vi "切换射频开关.vi"(8 "error in":errorcluster caption="error constant", 9 "COM":u16, 11 "A":u16) -> (0 "error out":errorcluster caption="error constant", 1 "ask":string, 2 "Isfailed":bool)   [LabVIEW 2015]
uses:
  Global/SeverGlobal.vi
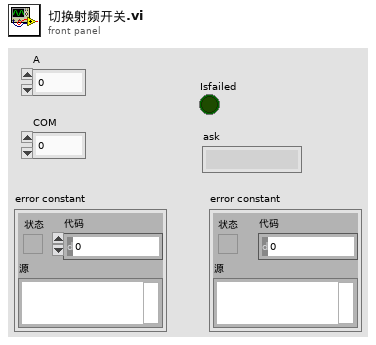
[diagram p1: front panel]
types:
  T1 = enum16{"Standard", "Buffered", "CRLF", "Immediate"}
  T2 = cluster{"IP_A":string, "PORT_A":i32, "IP_B":string, "PORT_B":i32, "IP_CLK":string, "PORT_CLK":i32, "IP_SWITCH":string, "PORT_SWITCH":i32}
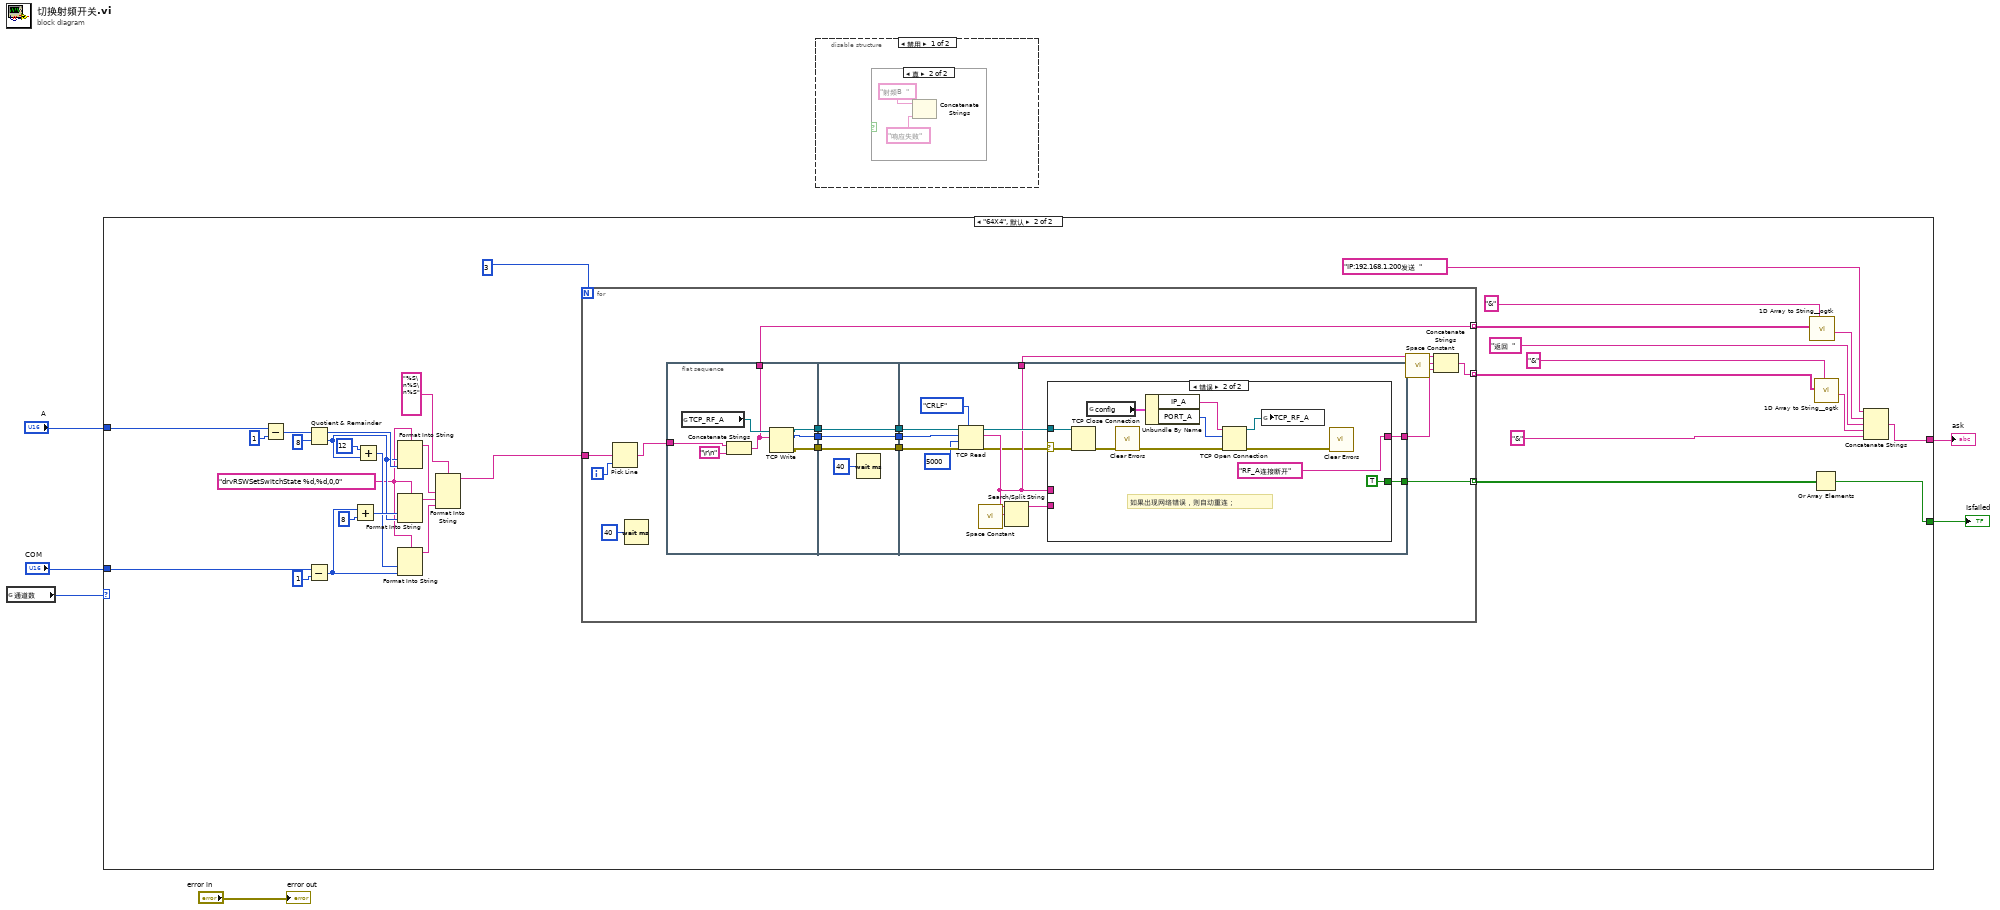
[diagram p0: block diagram]
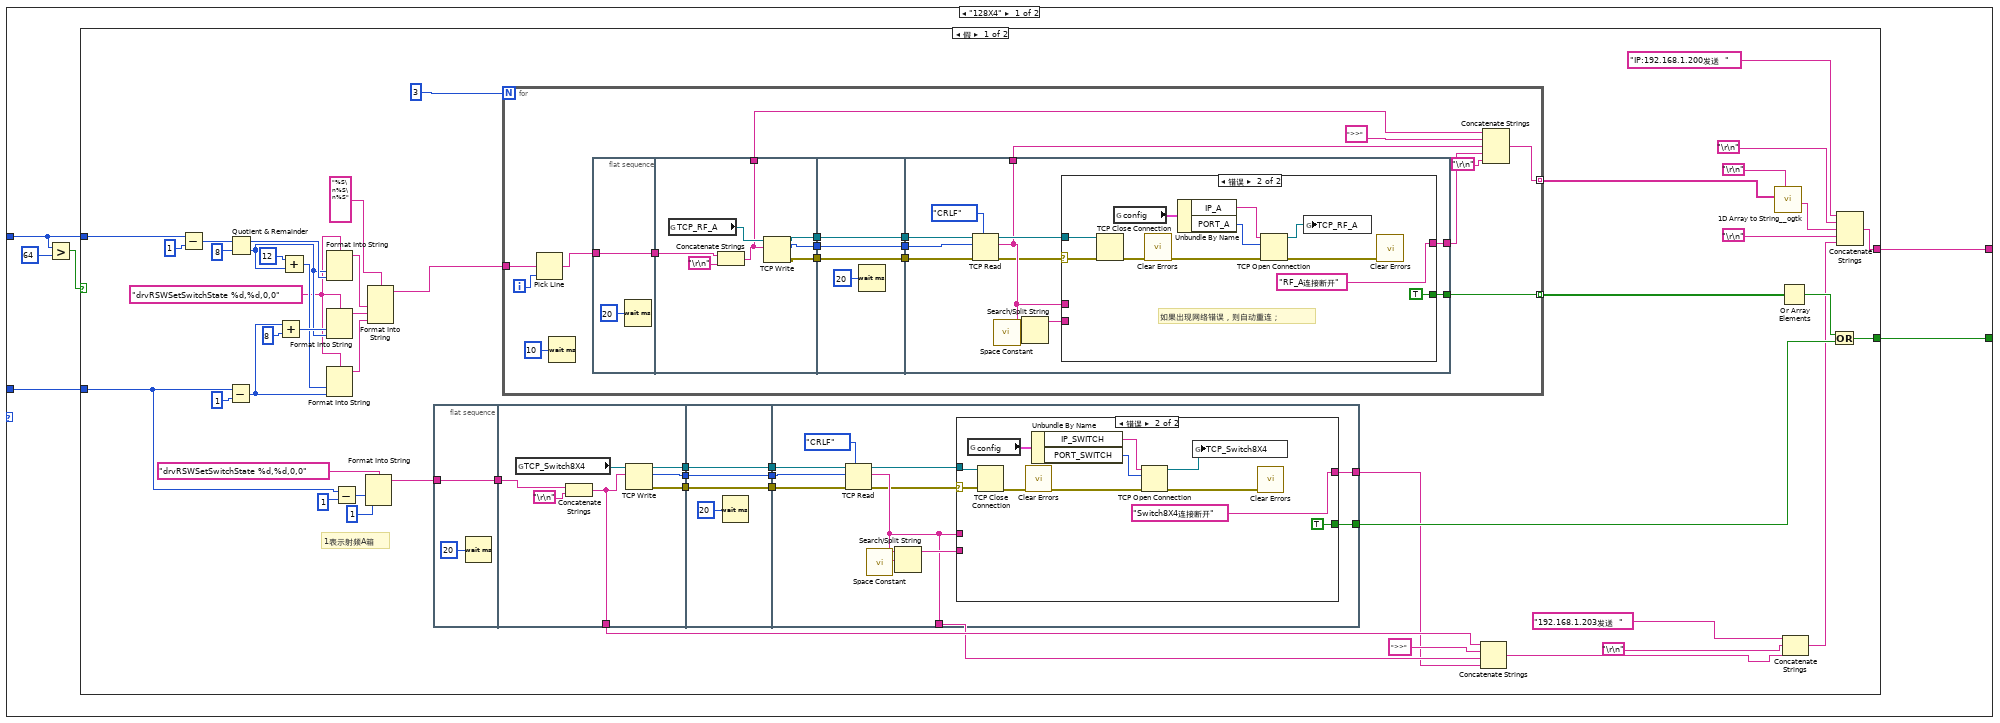
[diagram p2: hidden frame]
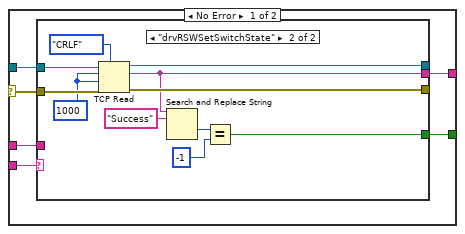
[diagram p3: hidden frame]
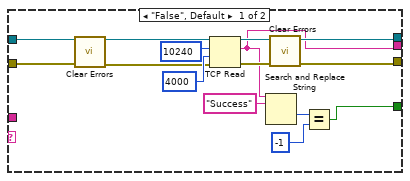
[diagram p4: hidden frame]
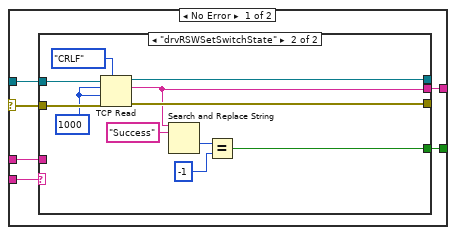
[diagram p5: hidden frame]
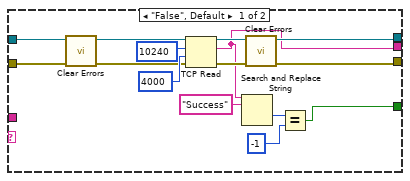
[diagram p6: hidden frame]
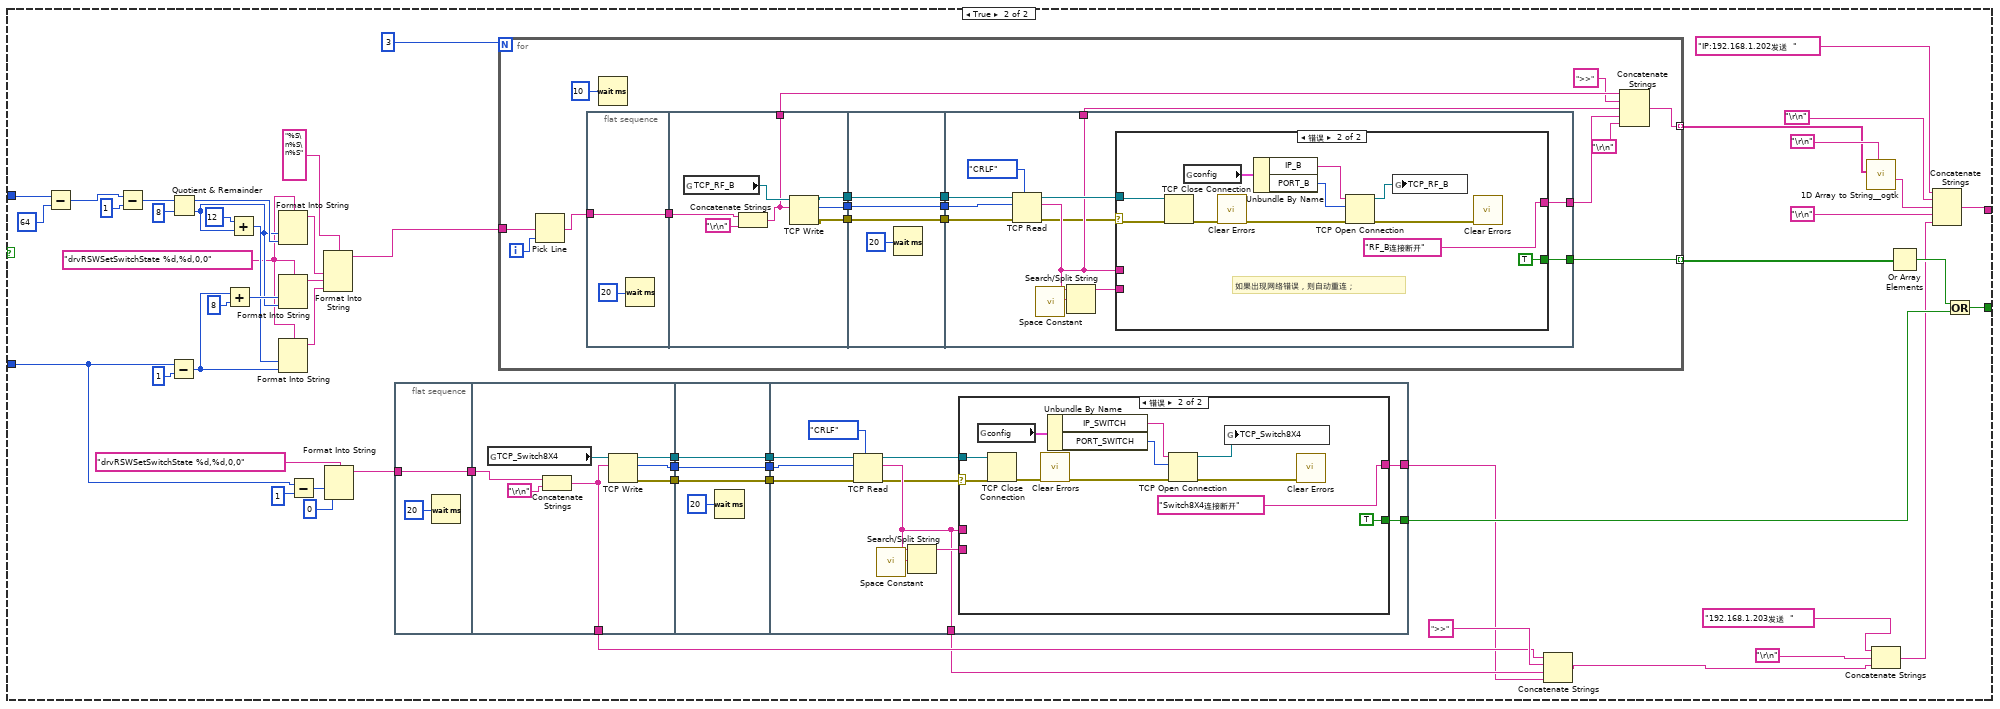
[diagram p7: hidden frame]
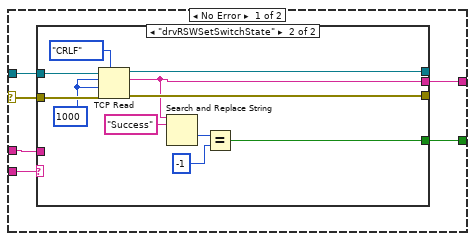
[diagram p8: hidden frame]
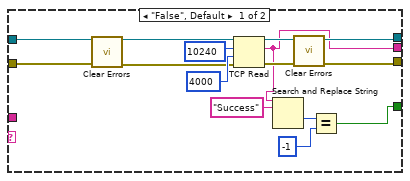
[diagram p9: hidden frame]
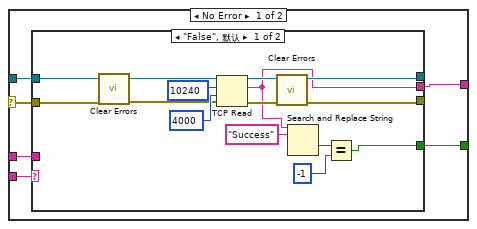
[diagram p10: hidden frame]
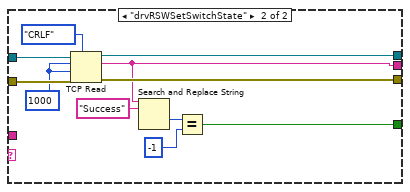
[diagram p11: hidden frame]
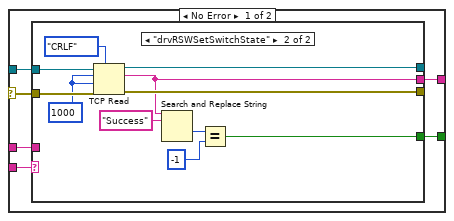
[diagram p12: hidden frame]
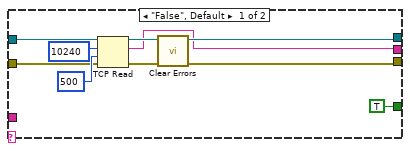
[diagram p13: hidden frame]
diagram:
  n1 = global read "SeverGlobal.vi" "通道数"() -> (w2:enum16{"64X4", "128X4"})
  n2 = case shown="\"64X4\", 默认" w2 {
    tunnel: "A" -> [w12 w444]
    tunnel: "COM" -> [w9 w443]
    tunnel: [w8 w423] -> w3
    tunnel: [w7 w413] -> w1
    frame "128X4" {
      n3 = Greater?(x=w12, y=u16 64) -> (0:w10:bool)
      n4 = case shown="假" w10 {
        tunnel: w12 -> [w45 w246]
        tunnel: w9 -> [w41 w232]
        tunnel: [w29 w229] -> w8
        tunnel: [w26 w218] -> w7
        frame False {
          w48 = "drvRSWSetSwitchState %d,%d,0,0" ("格式字符串")
          # "1表示射频A箱"
          n5 = Subtract(x=w45, y=1) -> (x-y=w62:i32)
          n6 = Subtract(x=w41, y=1) -> (x-y=w53:i32)
          n7 = Quotient & Remainder(x=w62, y=8) -> (x-y*floor(x/y)=w57:i32, floor(x/y)=w55:i32)
          n8 = Add(x=w53, y=8) -> (x+y=w56:i32)
          n9 = Add(x=12, y=w55) -> (x+y=w54:i32)
          n10 = Format Into String(format string=w48, w55, w57) -> (resulting string=w51:string)  [unwired: 2 in, 1 out]
          n11 = Format Into String(format string=w48, w56, w55) -> (resulting string=w50:string)  [unwired: 2 in, 1 out]
          n12 = Format Into String(format string=w48, w54, w53) -> (resulting string=w49:string)  [unwired: 2 in, 1 out]
          n13 = Subtract(x=w41, y=1) -> (x-y=w44:i32)
          n14 = Format Into String(format string="drvRSWSetSwitchState %d,%d,0,0" ("格式字符串"), w44, i16 1 ("input 2")) -> (resulting string=w39:string)  [unwired: 2 in, 1 out]
          n15 = Format Into String(format string="%S\n%S\n%S", w51, w50, w49) -> (resulting string=w47:string)  [unwired: 2 in, 1 out]
          n16 = flat-sequence {
            tunnel: w39 -> [w65]
            tunnel: [w65] -> w23
            tunnel: [w69] -> w38
            tunnel: [w68] -> w37
            tunnel: [w67] -> w33
            tunnel: [w66] -> w16
            tunnel: w23 -> [w71]
            tunnel: w38 -> [w75]
            tunnel: w37 -> [w74]
            tunnel: [w75] -> w36
            tunnel: [w74] -> w35
            tunnel: [w73] -> w34
            tunnel: w33 -> [w73]
            tunnel: w36 -> [w83]
            tunnel: w35 -> [w82]
            tunnel: w34 -> [w81]
            tunnel: [w80] -> w30
            tunnel: [w79] -> w14
            tunnel: [w78] -> w15
            frame #0 {
              n17 = Wait (ms)(milliseconds to wait=u32 20 ("delay")) -> ()  [unwired: 1 out]
            }
            frame #1 {
              n18 = global read "SeverGlobal.vi" "TCP_Switch8X4"() -> (w72:refnum<k5>)
              n19 = Concatenate Strings(w71, "\r\n") -> (w66:string)
              n20 = TCP Write(connection ID=w72, data in=w66) -> (connection ID out=w69:refnum<k5>, bytes written=w67:i32, error out=w68:errorcluster)  [unwired: 2 in]
            }
            frame #2 {
              n21 = Wait (ms)(milliseconds to wait=u32 20 ("delay")) -> ()  [unwired: 1 out]
            }
            frame #3 {
              n22 = TCP Read(connection ID=w83, bytes to read=w81, error in (no error)=w82, 7:T1."CRLF" ("mode (standard)")) -> (connection ID out=w87:refnum<k5>, data out=w78:string, error out=w77:errorcluster)  [unwired: 1 in]
              n23 = call <vilib>:"Space Constant.vi"() -> ("String"=w84:string)
              n24 = Search/Split String(string=w78, search string/char (-)=w84) -> (substring before match=w86:string)  [unwired: 1 in, 2 out]
              n25 = case shown="错误" w77 {
                selector: w77 -> [w88 w121]
                tunnel: w87 -> [w93 w120]
                tunnel: w86 -> [w92 _]
                tunnel: [w91 TRUE] -> w80
                tunnel: [w90 "Switch8X4连接断开" ("字符串")] -> w79
                tunnel: w78 -> [w89 _]
                frame No Error {
                  n26 = case shown="\"drvRSWSetSwitchState\"" w92 {
                    tunnel: [w102 w116] -> _
                    tunnel: [w101 w115] -> _
                    tunnel: w93 -> [w103 w114]
                    tunnel: w88 -> [w100 w113]
                    tunnel: w89 -> [_ _]
                    tunnel: [w94 w108] -> w91
                    tunnel: [w95 w107] -> w90
                    frame "False", Default {
                      n27 = call <vilib>:"Clear Errors.vi"("error in (no error)"=w100) -> ("error out"=w99:errorcluster)  [unwired: 5 in, 1 out]
                      n28 = TCP Read(connection ID=w103, bytes to read=10240, error in (no error)=w99, 9:4000 ("timeout ms (25000)")) -> (connection ID out=w102:refnum<k5>, data out=w95:string, error out=w105:errorcluster)  [unwired: 1 in]
                      n29 = Search and Replace String(input string=w95, search string="Success") -> (offset past replacement=w96:i32)  [unwired: 6 in, 3 out]
                      n30 = call <vilib>:"Clear Errors.vi"("error in (no error)"=w105) -> ("error out"=w101:errorcluster)  [unwired: 5 in, 1 out]
                      n31 = Equal?(x=w96, y=-1) -> (x = y?=w94:bool)
                    }
                    frame "drvRSWSetSwitchState" {
                      w112 = 1000 ("timeout ms (25000)")
                      n32 = TCP Read(connection ID=w114, bytes to read=w112, error in (no error)=w113, 7:T1."CRLF" ("mode (standard)"), 9:w112) -> (connection ID out=w116:refnum<k5>, data out=w107:string, error out=w115:errorcluster)
                      n33 = Search and Replace String(input string=w107, search string="Success") -> (offset past replacement=w110:i32)  [unwired: 6 in, 3 out]
                      n34 = Equal?(x=w110, y=-1) -> (x = y?=w108:bool)
                    }
                  }
                }
                frame Error {
                  n35 = global read "SeverGlobal.vi" "config"() -> (w124:T2)
                  n36 = TCP Close Connection(connection ID=w120, error in (no error)=w121) -> (error out=w122:errorcluster)  [unwired: 1 in, 1 out]
                  n37 = call <vilib>:"Clear Errors.vi"("error in (no error)"=w122) -> ("error out"=w123:errorcluster)  [unwired: 5 in, 1 out]
                  n38 = Unbundle By Name(w124) -> ("IP_SWITCH"=w125:string, "PORT_SWITCH"=w126:i32)
                  n39 = TCP Open Connection(address=w125, remote port or service name=w126, error in (no error)=w123) -> (connection ID=w127:refnum<k5>, error out=w128:errorcluster)  [unwired: 2 in]
                  n40 = global write "SeverGlobal.vi" "TCP_Switch8X4"(w127) -> ()
                  n41 = call <vilib>:"Clear Errors.vi"("error in (no error)"=w128) -> ()  [unwired: 5 in, 2 out]
                }
              }
            }
          }
          n42 = for {
            N: 3 -> [_]
            tunnel: w47 -> [w146]
            tunnel: [w136] -> w32 mode=indexing
            tunnel: [w133] -> w27 mode=indexing
            i -> [w145]
            n43 = Pick Line(multi-line string=w146, line index=w145) -> (output string=w144:string)  [unwired: 1 in]
            n44 = Wait (ms)(milliseconds to wait=u32 10 ("delay")) -> ()  [unwired: 1 out]
            n45 = flat-sequence {
              tunnel: w144 -> [w148]
              tunnel: [w148] -> w132
              tunnel: [w152] -> w142
              tunnel: [w151] -> w140
              tunnel: [w150] -> w138
              tunnel: [w149] -> w130
              tunnel: w132 -> [w153]
              tunnel: [w158] -> w143
              tunnel: w142 -> [w158]
              tunnel: [w157] -> w141
              tunnel: w140 -> [w157]
              tunnel: [w156] -> w139
              tunnel: w138 -> [w156]
              tunnel: w143 -> [w168]
              tunnel: w141 -> [w167]
              tunnel: w139 -> [w166]
              tunnel: [w163] -> w136
              tunnel: [w162] -> w135
              tunnel: [w161] -> w134
              frame #0 {
                n46 = Wait (ms)(milliseconds to wait=u32 20 ("delay")) -> ()  [unwired: 1 out]
              }
              frame #1 {
                n47 = global read "SeverGlobal.vi" "TCP_RF_A"() -> (w154:refnum<k5>)
                n48 = Concatenate Strings(w153, "\r\n") -> (w149:string)
                n49 = TCP Write(connection ID=w154, data in=w149) -> (connection ID out=w152:refnum<k5>, bytes written=w151:i32, error out=w150:errorcluster)  [unwired: 2 in]
              }
              frame #2 {
                n50 = Wait (ms)(milliseconds to wait=u32 20 ("delay")) -> ()  [unwired: 1 out]
              }
              frame #3 {
                n51 = TCP Read(connection ID=w168, bytes to read=w167, error in (no error)=w166, 7:T1."CRLF" ("mode (standard)")) -> (connection ID out=w164:refnum<k5>, data out=w162:string, error out=w160:errorcluster)  [unwired: 1 in]
                n52 = call <vilib>:"Space Constant.vi"() -> ("String"=w170:string)
                n53 = Search/Split String(string=w162, search string/char (-)=w170) -> (substring before match=w165:string)  [unwired: 1 in, 2 out]
                n54 = case shown="错误" w160 {
                  selector: w160 -> [w171 w210]
                  tunnel: w165 -> [w176 _]
                  tunnel: w164 -> [w175 w211]
                  tunnel: [w174 TRUE] -> w163
                  tunnel: w162 -> [w173 _]
                  tunnel: [w172 "RF_A连接断开" ("字符串")] -> w161
                  frame No Error {
                    n55 = case shown="\"drvRSWSetSwitchState\"" w176 {
                      tunnel: [w185 w199] -> _
                      tunnel: [w184 w198] -> _
                      tunnel: w175 -> [w186 w197]
                      tunnel: w171 -> [w183 w196]
                      tunnel: w173 -> [_ _]
                      tunnel: [w177 w191] -> w174
                      tunnel: [w178 w190] -> w172
                      frame "False", Default {
                        n56 = call <vilib>:"Clear Errors.vi"("error in (no error)"=w183) -> ("error out"=w182:errorcluster)  [unwired: 5 in, 1 out]
                        n57 = TCP Read(connection ID=w186, bytes to read=10240, error in (no error)=w182, 9:4000 ("timeout ms (25000)")) -> (connection ID out=w185:refnum<k5>, data out=w178:string, error out=w188:errorcluster)  [unwired: 1 in]
                        n58 = Search and Replace String(input string=w178, search string="Success") -> (offset past replacement=w181:i32)  [unwired: 6 in, 3 out]
                        n59 = call <vilib>:"Clear Errors.vi"("error in (no error)"=w188) -> ("error out"=w184:errorcluster)  [unwired: 5 in, 1 out]
                        n60 = Equal?(x=w181, y=-1) -> (x = y?=w177:bool)
                      }
                      frame "drvRSWSetSwitchState" {
                        w195 = 1000 ("timeout ms (25000)")
                        n61 = TCP Read(connection ID=w197, bytes to read=w195, error in (no error)=w196, 7:T1."CRLF" ("mode (standard)"), 9:w195) -> (connection ID out=w199:refnum<k5>, data out=w190:string, error out=w198:errorcluster)
                        n62 = Search and Replace String(input string=w190, search string="Success") -> (offset past replacement=w193:i32)  [unwired: 6 in, 3 out]
                        n63 = Equal?(x=w193, y=-1) -> (x = y?=w191:bool)
                      }
                    }
                  }
                  frame Error {
                    # "如果出现网络错误，则自动重连；"
                    n64 = TCP Close Connection(connection ID=w211, error in (no error)=w210) -> (error out=w209:errorcluster)  [unwired: 1 in, 1 out]
                    n65 = global read "SeverGlobal.vi" "config"() -> (w207:T2)
                    n66 = call <vilib>:"Clear Errors.vi"("error in (no error)"=w209) -> ("error out"=w208:errorcluster)  [unwired: 5 in, 1 out]
                    n67 = Unbundle By Name(w207) -> ("IP_A"=w206:string, "PORT_A"=w205:i32)
                    n68 = TCP Open Connection(address=w206, remote port or service name=w205, error in (no error)=w208) -> (connection ID=w204:refnum<k5>, error out=w203:errorcluster)  [unwired: 2 in]
                    n69 = global write "SeverGlobal.vi" "TCP_RF_A"(w204) -> ()
                    n70 = call <vilib>:"Clear Errors.vi"("error in (no error)"=w203) -> ()  [unwired: 5 in, 2 out]
                  }
                }
              }
            }
            n71 = Concatenate Strings(w130, ">>" ("字符串"), w135, w134, "\r\n") -> (w133:string)
          }
          n72 = Concatenate Strings(w16, ">>" ("字符串"), w15, w14) -> (w13:string)
          n73 = call <userlib>:"1D Array to String__ogtk.vi"("delimiter (Tab)"="\r\n", "Array of Strings"=w27) -> ("delimited string"=w28:string)  [unwired: 9 in]
          n74 = Or Array Elements(Boolean array=w32) -> (logical OR=w31:bool)
          n75 = Concatenate Strings("192.168.1.203发送  " ("delimiter (Tab)"), "\r\n", w13) -> (w24:string)
          n76 = Or(x=w31, y=w30) -> (x .or. y?=w29:bool)
          n77 = Concatenate Strings("IP:192.168.1.200发送  " ("delimiter (Tab)"), "\r\n", w28, "\r\n", w24) -> (w26:string)
        }
        frame True {
          w249 = "drvRSWSetSwitchState %d,%d,0,0" ("格式字符串")
          n78 = Subtract(x=w246, y=u16 64) -> (x-y=w244:u16)
          n79 = Subtract(x=w244, y=1) -> (x-y=w263:i32)
          n80 = Subtract(x=w232, y=1) -> (x-y=w254:i32)
          n81 = Quotient & Remainder(x=w263, y=8) -> (x-y*floor(x/y)=w258:i32, floor(x/y)=w256:i32)
          n82 = Add(x=w254, y=8) -> (x+y=w257:i32)
          n83 = Add(x=12, y=w256) -> (x+y=w255:i32)
          n84 = Format Into String(format string=w249, w256, w258) -> (resulting string=w252:string)  [unwired: 2 in, 1 out]
          n85 = Format Into String(format string=w249, w257, w256) -> (resulting string=w251:string)  [unwired: 2 in, 1 out]
          n86 = Format Into String(format string=w249, w255, w254) -> (resulting string=w250:string)  [unwired: 2 in, 1 out]
          n87 = Subtract(x=w232, y=1) -> (x-y=w237:i32)
          n88 = Format Into String(format string="%S\n%S\n%S", w252, w251, w250) -> (resulting string=w248:string)  [unwired: 2 in, 1 out]
          n89 = Format Into String(format string="drvRSWSetSwitchState %d,%d,0,0" ("格式字符串"), w237, i16 0 ("input 2")) -> (resulting string=w233:string)  [unwired: 2 in, 1 out]
          n90 = flat-sequence {
            tunnel: w233 -> [w266]
            tunnel: [w266] -> w226
            tunnel: [w270] -> w243
            tunnel: [w269] -> w242
            tunnel: [w268] -> w241
            tunnel: [w267] -> w216
            tunnel: w226 -> [w272]
            tunnel: w243 -> [w276]
            tunnel: w242 -> [w275]
            tunnel: [w276] -> w240
            tunnel: [w275] -> w239
            tunnel: [w274] -> w238
            tunnel: w241 -> [w274]
            tunnel: w240 -> [w284]
            tunnel: w239 -> [w283]
            tunnel: w238 -> [w282]
            tunnel: [w281] -> w228
            tunnel: [w280] -> w215
            tunnel: [w279] -> w214
            frame #0 {
              n91 = Wait (ms)(milliseconds to wait=u32 20 ("delay")) -> ()  [unwired: 1 out]
            }
            frame #1 {
              n92 = global read "SeverGlobal.vi" "TCP_Switch8X4"() -> (w273:refnum<k5>)
              n93 = Concatenate Strings(w272, "\r\n") -> (w267:string)
              n94 = TCP Write(connection ID=w273, data in=w267) -> (connection ID out=w270:refnum<k5>, bytes written=w268:i32, error out=w269:errorcluster)  [unwired: 2 in]
            }
            frame #2 {
              n95 = Wait (ms)(milliseconds to wait=u32 20 ("delay")) -> ()  [unwired: 1 out]
            }
            frame #3 {
              n96 = TCP Read(connection ID=w284, bytes to read=w282, error in (no error)=w283, 7:T1."CRLF" ("mode (standard)")) -> (connection ID out=w288:refnum<k5>, data out=w280:string, error out=w278:errorcluster)  [unwired: 1 in]
              n97 = call <vilib>:"Space Constant.vi"() -> ("String"=w285:string)
              n98 = Search/Split String(string=w280, search string/char (-)=w285) -> (substring before match=w287:string)  [unwired: 1 in, 2 out]
              n99 = case shown="错误" w278 {
                selector: w278 -> [w289 w322]
                tunnel: w288 -> [w294 w321]
                tunnel: w287 -> [w293 _]
                tunnel: [w292 TRUE] -> w281
                tunnel: w280 -> [w291 _]
                tunnel: [w290 "Switch8X4连接断开" ("字符串")] -> w279
                frame No Error {
                  n100 = case shown="\"drvRSWSetSwitchState\"" w293 {
                    tunnel: [w303 w317] -> _
                    tunnel: [w302 w316] -> _
                    tunnel: w294 -> [w304 w315]
                    tunnel: w289 -> [w301 w314]
                    tunnel: w291 -> [_ _]
                    tunnel: [w295 w309] -> w292
                    tunnel: [w297 w308] -> w290
                    frame "False", Default {
                      n101 = call <vilib>:"Clear Errors.vi"("error in (no error)"=w301) -> ("error out"=w300:errorcluster)  [unwired: 5 in, 1 out]
                      n102 = TCP Read(connection ID=w304, bytes to read=10240, error in (no error)=w300, 9:4000 ("timeout ms (25000)")) -> (connection ID out=w303:refnum<k5>, data out=w297:string, error out=w306:errorcluster)  [unwired: 1 in]
                      n103 = Search and Replace String(input string=w297, search string="Success") -> (offset past replacement=w298:i32)  [unwired: 6 in, 3 out]
                      n104 = call <vilib>:"Clear Errors.vi"("error in (no error)"=w306) -> ("error out"=w302:errorcluster)  [unwired: 5 in, 1 out]
                      n105 = Equal?(x=w298, y=-1) -> (x = y?=w295:bool)
                    }
                    frame "drvRSWSetSwitchState" {
                      w313 = 1000 ("timeout ms (25000)")
                      n106 = TCP Read(connection ID=w315, bytes to read=w313, error in (no error)=w314, 7:T1."CRLF" ("mode (standard)"), 9:w313) -> (connection ID out=w317:refnum<k5>, data out=w308:string, error out=w316:errorcluster)
                      n107 = Search and Replace String(input string=w308, search string="Success") -> (offset past replacement=w311:i32)  [unwired: 6 in, 3 out]
                      n108 = Equal?(x=w311, y=-1) -> (x = y?=w309:bool)
                    }
                  }
                }
                frame Error {
                  n109 = global read "SeverGlobal.vi" "config"() -> (w325:T2)
                  n110 = TCP Close Connection(connection ID=w321, error in (no error)=w322) -> (error out=w323:errorcluster)  [unwired: 1 in, 1 out]
                  n111 = call <vilib>:"Clear Errors.vi"("error in (no error)"=w323) -> ("error out"=w324:errorcluster)  [unwired: 5 in, 1 out]
                  n112 = Unbundle By Name(w325) -> ("IP_SWITCH"=w326:string, "PORT_SWITCH"=w327:i32)
                  n113 = TCP Open Connection(address=w326, remote port or service name=w327, error in (no error)=w324) -> (connection ID=w328:refnum<k5>, error out=w329:errorcluster)  [unwired: 2 in]
                  n114 = global write "SeverGlobal.vi" "TCP_Switch8X4"(w328) -> ()
                  n115 = call <vilib>:"Clear Errors.vi"("error in (no error)"=w329) -> ()  [unwired: 5 in, 2 out]
                }
              }
            }
          }
          n116 = for {
            N: 3 -> [_]
            tunnel: w248 -> [w347]
            tunnel: [w338] -> w230 mode=indexing
            tunnel: [w330] -> w220 mode=indexing
            i -> [w346]
            n117 = Pick Line(multi-line string=w347, line index=w346) -> (output string=w345:string)  [unwired: 1 in]
            n118 = flat-sequence {
              tunnel: w345 -> [w349]
              tunnel: [w349] -> w337
              tunnel: [w353] -> w343
              tunnel: [w352] -> w341
              tunnel: [w351] -> w339
              tunnel: [w350] -> w334
              tunnel: w337 -> [w354]
              tunnel: [w359] -> w344
              tunnel: w343 -> [w359]
              tunnel: [w358] -> w342
              tunnel: w341 -> [w358]
              tunnel: [w357] -> w340
              tunnel: w339 -> [w357]
              tunnel: w344 -> [w369]
              tunnel: w342 -> [w368]
              tunnel: w340 -> [w367]
              tunnel: [w364] -> w338
              tunnel: [w363] -> w332
              tunnel: [w362] -> w331
              frame #0 {
                n119 = Wait (ms)(milliseconds to wait=u32 20 ("delay")) -> ()  [unwired: 1 out]
              }
              frame #1 {
                n120 = global read "SeverGlobal.vi" "TCP_RF_B"() -> (w355:refnum<k5>)
                n121 = Concatenate Strings(w354, "\r\n") -> (w350:string)
                n122 = TCP Write(connection ID=w355, data in=w350) -> (connection ID out=w353:refnum<k5>, bytes written=w352:i32, error out=w351:errorcluster)  [unwired: 2 in]
              }
              frame #2 {
                n123 = Wait (ms)(milliseconds to wait=u32 20 ("delay")) -> ()  [unwired: 1 out]
              }
              frame #3 {
                n124 = TCP Read(connection ID=w369, bytes to read=w368, error in (no error)=w367, 7:T1."CRLF" ("mode (standard)")) -> (connection ID out=w365:refnum<k5>, data out=w363:string, error out=w361:errorcluster)  [unwired: 1 in]
                n125 = call <vilib>:"Space Constant.vi"() -> ("String"=w371:string)
                n126 = Search/Split String(string=w363, search string/char (-)=w371) -> (substring before match=w366:string)  [unwired: 1 in, 2 out]
                n127 = case shown="错误" w361 {
                  selector: w361 -> [w372 w405]
                  tunnel: w366 -> [w377 _]
                  tunnel: w365 -> [w376 w404]
                  tunnel: [w375 TRUE] -> w364
                  tunnel: w363 -> [w374 _]
                  tunnel: [w373 "RF_B连接断开" ("字符串")] -> w362
                  frame No Error {
                    n128 = case shown="\"False\", 默认" w377 {
                      tunnel: [w386 w400] -> _
                      tunnel: [w385 w399] -> _
                      tunnel: w376 -> [w387 w398]
                      tunnel: w372 -> [w384 w397]
                      tunnel: w374 -> [_ _]
                      tunnel: [w378 w392] -> w375
                      tunnel: [w379 w391] -> w373
                      frame "False", Default {
                        n129 = call <vilib>:"Clear Errors.vi"("error in (no error)"=w384) -> ("error out"=w383:errorcluster)  [unwired: 5 in, 1 out]
                        n130 = TCP Read(connection ID=w387, bytes to read=10240, error in (no error)=w383, 9:4000 ("timeout ms (25000)")) -> (connection ID out=w386:refnum<k5>, data out=w379:string, error out=w389:errorcluster)  [unwired: 1 in]
                        n131 = call <vilib>:"Clear Errors.vi"("error in (no error)"=w389) -> ("error out"=w385:errorcluster)  [unwired: 5 in, 1 out]
                        n132 = Search and Replace String(input string=w379, search string="Success") -> (offset past replacement=w381:i32)  [unwired: 6 in, 3 out]
                        n133 = Equal?(x=w381, y=-1) -> (x = y?=w378:bool)
                      }
                      frame "drvRSWSetSwitchState" {
                        w396 = 1000 ("timeout ms (25000)")
                        n134 = TCP Read(connection ID=w398, bytes to read=w396, error in (no error)=w397, 7:T1."CRLF" ("mode (standard)"), 9:w396) -> (connection ID out=w400:refnum<k5>, data out=w391:string, error out=w399:errorcluster)
                        n135 = Search and Replace String(input string=w391, search string="Success") -> (offset past replacement=w394:i32)  [unwired: 6 in, 3 out]
                        n136 = Equal?(x=w394, y=-1) -> (x = y?=w392:bool)
                      }
                    }
                  }
                  frame Error {
                    # "如果出现网络错误，则自动重连；"
                    n137 = TCP Close Connection(connection ID=w404, error in (no error)=w405) -> (error out=w406:errorcluster)  [unwired: 1 in, 1 out]
                    n138 = global read "SeverGlobal.vi" "config"() -> (w408:T2)
                    n139 = call <vilib>:"Clear Errors.vi"("error in (no error)"=w406) -> ("error out"=w407:errorcluster)  [unwired: 5 in, 1 out]
                    n140 = Unbundle By Name(w408) -> ("IP_B"=w409:string, "PORT_B"=w410:i32)
                    n141 = TCP Open Connection(address=w409, remote port or service name=w410, error in (no error)=w407) -> (connection ID=w411:refnum<k5>, error out=w412:errorcluster)  [unwired: 2 in]
                    n142 = global write "SeverGlobal.vi" "TCP_RF_B"(w411) -> ()
                    n143 = call <vilib>:"Clear Errors.vi"("error in (no error)"=w412) -> ()  [unwired: 5 in, 2 out]
                  }
                }
              }
            }
            n144 = Wait (ms)(milliseconds to wait=u32 10 ("delay")) -> ()  [unwired: 1 out]
            n145 = Concatenate Strings(w334, ">>" ("字符串"), w332, w331, "\r\n") -> (w330:string)
          }
          n146 = Concatenate Strings(w216, ">>" ("字符串"), w215, w214) -> (w212:string)
          n147 = call <userlib>:"1D Array to String__ogtk.vi"("delimiter (Tab)"="\r\n", "Array of Strings"=w220) -> ("delimited string"=w225:string)  [unwired: 9 in]
          n148 = Concatenate Strings("192.168.1.203发送  " ("delimiter (Tab)"), "\r\n", w212) -> (w219:string)
          n149 = Or Array Elements(Boolean array=w230) -> (logical OR=w231:bool)
          n150 = Concatenate Strings("IP:192.168.1.202发送  " ("delimiter (Tab)"), "\r\n", w225, "\r\n", w219) -> (w218:string)
          n151 = Or(x=w231, y=w228) -> (x .or. y?=w229:bool)
        }
      }
    }
    frame "64X4", Default {
      w427 = "drvRSWSetSwitchState %d,%d,0,0" ("格式字符串")
      n152 = Subtract(x=w444, y=1) -> (x-y=w441:i32)
      n153 = Subtract(x=w443, y=1) -> (x-y=w432:i32)
      n154 = Quotient & Remainder(x=w441, y=8) -> (x-y*floor(x/y)=w436:i32, floor(x/y)=w434:i32)
      n155 = Add(x=w432, y=8) -> (x+y=w435:i32)
      n156 = Add(x=12, y=w434) -> (x+y=w433:i32)
      n157 = Format Into String(format string=w427, w434, w436) -> (resulting string=w430:string)  [unwired: 2 in, 1 out]
      n158 = Format Into String(format string=w427, w435, w434) -> (resulting string=w429:string)  [unwired: 2 in, 1 out]
      n159 = Format Into String(format string=w427, w433, w432) -> (resulting string=w428:string)  [unwired: 2 in, 1 out]
      n160 = Format Into String(format string="%S\n%S\n%S", w430, w429, w428) -> (resulting string=w426:string)  [unwired: 2 in, 1 out]
      n161 = for {
        N: 3 -> [_]
        tunnel: w426 -> [w460]
        tunnel: [w450] -> w424 mode=indexing
        tunnel: [w449] -> w415 mode=indexing
        tunnel: [w445] -> w414 mode=indexing
        i -> [w459]
        n162 = Pick Line(multi-line string=w460, line index=w459) -> (output string=w458:string)  [unwired: 1 in]
        n163 = Wait (ms)(milliseconds to wait=u32 40 ("delay")) -> ()  [unwired: 1 out]
        n164 = flat-sequence {
          tunnel: w458 -> [w465]
          tunnel: [w464] -> w456
          tunnel: [w463] -> w454
          tunnel: [w462] -> w452
          tunnel: [w461] -> w449
          tunnel: [w470] -> w457
          tunnel: w456 -> [w470]
          tunnel: [w469] -> w455
          tunnel: w454 -> [w469]
          tunnel: [w468] -> w453
          tunnel: w452 -> [w468]
          tunnel: w457 -> [w481]
          tunnel: w455 -> [w480]
          tunnel: w453 -> [w479]
          tunnel: [w475] -> w450
          tunnel: [w474] -> w448
          tunnel: [w473] -> w446
          frame #0 {
            n165 = global read "SeverGlobal.vi" "TCP_RF_A"() -> (w466:refnum<k5>)
            n166 = Concatenate Strings(w465, "\r\n") -> (w461:string)
            n167 = TCP Write(connection ID=w466, data in=w461) -> (connection ID out=w464:refnum<k5>, bytes written=w463:i32, error out=w462:errorcluster)  [unwired: 2 in]
          }
          frame #1 {
            n168 = Wait (ms)(milliseconds to wait=u32 40 ("delay")) -> ()  [unwired: 1 out]
          }
          frame #2 {
            n169 = TCP Read(connection ID=w481, bytes to read=w480, error in (no error)=w479, 7:T1."CRLF" ("mode (standard)"), 9:5000 ("timeout ms (25000)")) -> (connection ID out=w476:refnum<k5>, data out=w474:string, error out=w472:errorcluster)
            n170 = call <vilib>:"Space Constant.vi"() -> ("String"=w483:string)
            n171 = Search/Split String(string=w474, search string/char (-)=w483) -> (substring before match=w477:string)  [unwired: 1 in, 2 out]
            n172 = case shown="错误" w472 {
              selector: w472 -> [w484 w513]
              tunnel: w477 -> [w489 _]
              tunnel: w476 -> [w488 w512]
              tunnel: [w487 TRUE] -> w475
              tunnel: w474 -> [w486 _]
              tunnel: [w485 "RF_A连接断开" ("字符串")] -> w473
              frame No Error {
                n173 = case shown="\"drvRSWSetSwitchState\"" w489 {
                  tunnel: [w493 w508] -> _
                  tunnel: [w492 w507] -> _
                  tunnel: w488 -> [w495 w506]
                  tunnel: w484 -> [w494 w505]
                  tunnel: w486 -> [_ _]
                  tunnel: [TRUE w500] -> w487
                  tunnel: [w490 w499] -> w485
                  frame "False", Default {
                    n174 = TCP Read(connection ID=w495, bytes to read=10240, error in (no error)=w494, 9:500 ("timeout ms (25000)")) -> (connection ID out=w493:refnum<k5>, data out=w490:string, error out=w497:errorcluster)  [unwired: 1 in]
                    n175 = call <vilib>:"Clear Errors.vi"("error in (no error)"=w497) -> ("error out"=w492:errorcluster)  [unwired: 5 in, 1 out]
                  }
                  frame "drvRSWSetSwitchState" {
                    w504 = 1000 ("timeout ms (25000)")
                    n176 = TCP Read(connection ID=w506, bytes to read=w504, error in (no error)=w505, 7:T1."CRLF" ("mode (standard)"), 9:w504) -> (connection ID out=w508:refnum<k5>, data out=w499:string, error out=w507:errorcluster)
                    n177 = Search and Replace String(input string=w499, search string="Success") -> (offset past replacement=w502:i32)  [unwired: 6 in, 3 out]
                    n178 = Equal?(x=w502, y=-1) -> (x = y?=w500:bool)
                  }
                }
              }
              frame Error {
                # "如果出现网络错误，则自动重连；"
                n179 = TCP Close Connection(connection ID=w512, error in (no error)=w513) -> (error out=w520:errorcluster)  [unwired: 1 in, 1 out]
                n180 = global read "SeverGlobal.vi" "config"() -> (w518:T2)
                n181 = call <vilib>:"Clear Errors.vi"("error in (no error)"=w520) -> ("error out"=w519:errorcluster)  [unwired: 5 in, 1 out]
                n182 = Unbundle By Name(w518) -> ("IP_A"=w517:string, "PORT_A"=w516:i32)
                n183 = TCP Open Connection(address=w517, remote port or service name=w516, error in (no error)=w519) -> (connection ID=w515:refnum<k5>, error out=w514:errorcluster)  [unwired: 2 in]
                n184 = global write "SeverGlobal.vi" "TCP_RF_A"(w515) -> ()
                n185 = call <vilib>:"Clear Errors.vi"("error in (no error)"=w514) -> ()  [unwired: 5 in, 2 out]
              }
            }
          }
        }
        n186 = call <vilib>:"Space Constant.vi"() -> ("String"=w447:string)
        n187 = Concatenate Strings(w448, w447, w446) -> (w445:string)
      }
      n188 = call <userlib>:"1D Array to String__ogtk.vi"("delimiter (Tab)"="&", "Array of Strings"=w415) -> ("delimited string"=w417:string)  [unwired: 9 in]
      n189 = Or Array Elements(Boolean array=w424) -> (logical OR=w423:bool)
      n190 = call <userlib>:"1D Array to String__ogtk.vi"("delimiter (Tab)"="&", "Array of Strings"=w414) -> ("delimited string"=w421:string)  [unwired: 9 in]
      n191 = Concatenate Strings("IP:192.168.1.200发送  " ("delimiter (Tab)"), w417, "返回  " ("字符串"), w421, "&" ("delimiter (Tab)")) -> (w413:string)
    }
  }
  "Isfailed" <- w3
  "ask" <- w1
  n192 = disable-structure shown="禁用" {
    frame Disabled {
      n193 = case shown="真" {
        selector: _ -> [_ _]
        frame False {
        }
        frame True {
          n194 = Concatenate Strings("射频B  " ("message"), "响应失败" ("message")) -> (w523:string)  [unwired: 1 out]
        }
      }
    }
    frame Enabled {
    }
  }
  "error out" <- "error in"
